vi "Run Automatic Tests.vi"() -> ()   [LabVIEW 2017, in "Unit Tests.lvlib"]
uses:
  Unit Tests.lvlib
panel:
  in  "# of runs":i32=3
  out "error out":errorcluster
  in  "error in (no error)":errorcluster
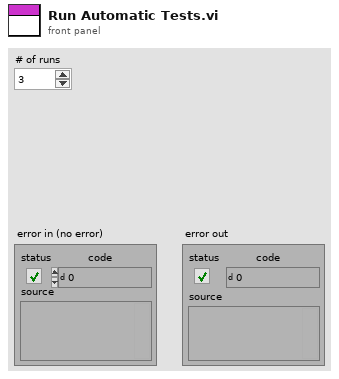
[diagram p1: front panel]
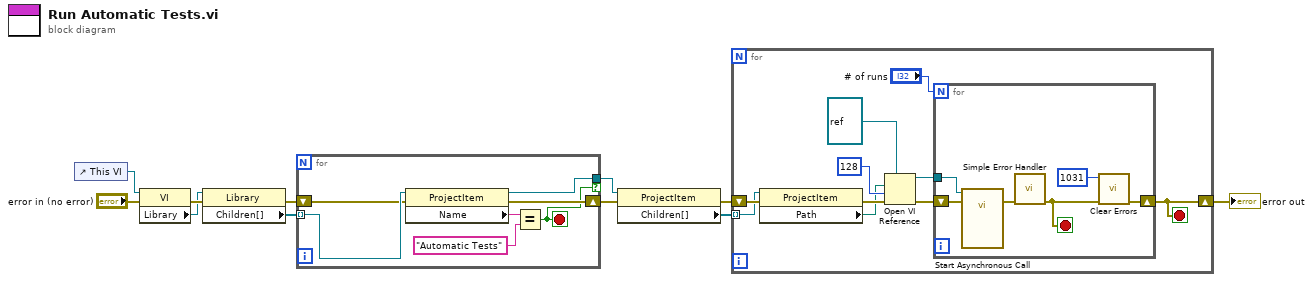
[diagram p0: block diagram]
diagram:
  n1 = control-ref of="This VI"() -> (w11:refnum<vi>)
  n2 = property class="VI"(reference=w11, error in="error in (no error)") -> (error out=w6:errorcluster, "Library"=w1:refnum<vi>)  [unwired: 1 out]
  n3 = property class="Library"(reference=w1, error in=w6) -> (error out=w5:errorcluster, "Children[]"=w10:refnum<vi>[])  [unwired: 1 out]
  n4 = for {
    tunnel: w10 -> [w18] mode=indexing
    tunnel: [w15] -> w9 if=w12
    shift-right: [w13] -> w4
    shift-left: w5 -> [w14]
    stop <- w12 stop-if-true
    n5 = property class="ProjectItem"(reference=w18, error in=w14) -> (reference out=w15:refnum<vi>, error out=w13:errorcluster, "Name"=w17:string)
    n6 = Equal?(x=w17, y="Automatic Tests") -> (x = y?=w12:bool)
  }
  n7 = property class="ProjectItem"(reference=w9, error in=w4) -> (error out=w3:errorcluster, "Children[]"=w8:refnum<vi>[])  [unwired: 1 out]
  n8 = for {
    tunnel: w8 -> [w21] mode=indexing
    shift-right: [w19] -> w2
    shift-left: w3 -> [w22]
    stop <- w19 stop-if-true
    n9 = property class="ProjectItem"(reference=w21, error in=w22) -> (error out=w26:errorcluster, "Path"=w20:path)  [unwired: 1 out]
    n10 = Open VI Reference(type specifier VI Refnum (for type only)=refnum<vi> refnum, vi path=w20, options=128, error in (no error)=w26) -> (vi reference=w27:refnum<vi>, error out=w25:errorcluster)  [unwired: 2 in]
    n11 = for {
      N: "# of runs" -> [_]
      tunnel: w27 -> [w34]
      shift-right: [w31] -> w19
      shift-left: w25 -> [w33]
      stop <- w29 stop-if-true
      n12 = call-by-ref "Start Asynchronous Call"(reference=w34, error in=w33) -> (error out=w32:errorcluster)  [unwired: 11 in, 2 out]
      n13 = call <vilib>:"Simple Error Handler.vi"("error in (no error)"=w32) -> ("error out"=w29:errorcluster)  [unwired: 4 in, 4 out]
      n14 = call <vilib>:"Clear Errors.vi"("error in (no error)"=w29, "specific error code to clear (0: all)"=1031) -> ("error out"=w31:errorcluster)  [unwired: 4 in, 1 out]
    }
  }
  "error out" <- w2
